vi "RescaleSpectrometerGraph.vi"(10 "Previous Ymax":dbl, 11 "Array":T1(array[cluster])) -> (3 "Ymax":dbl)   [LabVIEW 2012]
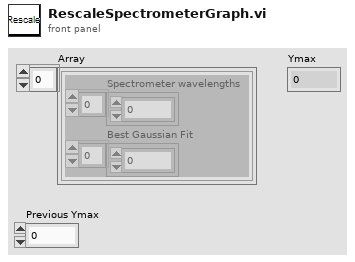
[diagram p1: front panel]
types:
  T1 = cluster{"Spectrometer wavelengths":sgl[], "Best Gaussian Fit":dbl[]}[]
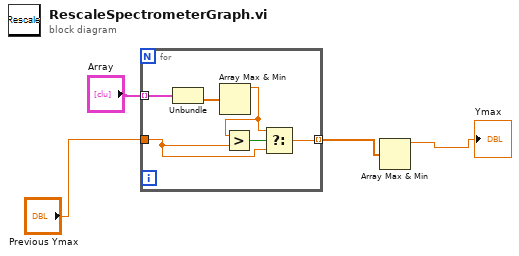
[diagram p0: block diagram]
diagram:
  n1 = for {
    tunnel: "Array" -> [w10] mode=indexing
    tunnel: "Previous Ymax" -> [w5]
    tunnel: [w7] -> w2 mode=indexing
    n2 = Unbundle(w10) -> ("Best Gaussian Fit"=w9:dbl[])  [unwired: 1 out]
    n3 = Array Max & Min(array=w9) -> (max value=w6:dbl)  [unwired: 3 out]
    n4 = Greater?(x=w6, y=w5) -> (0:w8:bool)
    n5 = Select(t=w6, s=w8, f=w5) -> (s? t:f=w7:dbl)
  }
  n6 = Array Max & Min(array=w2) -> (max value=→"Ymax":dbl)  [unwired: 3 out]
